vi "RXMux-Remote.vi"() -> ()   [LabVIEW 2009]
uses:
  <vilib>/NXT/Subs/LVHSConnector.ctl
  <vilib>/NXT/Block Support/NXT_InputPort.ctl
  <vilib>/NXT/Dual Mode Library/Display/drawNumber.vi
  <vilib>/NXT/Dual Mode Library/Display/drawText.vi
panel:
  in  "Channe to  Select":u8(ring) items=["Read Channel", "Select Ch1", "Select Ch2", "Select Ch3", "Select Ch4"]
  out "NXT dup":T1
  in  "Input Port":T2 items=["Port 1", "Port 2", "Port 3", "Port 4"]
  in  "stop":bool
  in  "NXT":T1
  # "mindsensors.com\nCopyright (c) 2009 by mindsensors.com\nEmail: info (<at>) mindsensors (<dot>) com\n\nThis program is free software. You can redistribute it and/or modify\nit under the terms of the GNU General Public License as published by\nthe Free Software Foundation; version 3 of the License.\nRead the license at: http://www.gnu.org/licenses/gpl.txt"
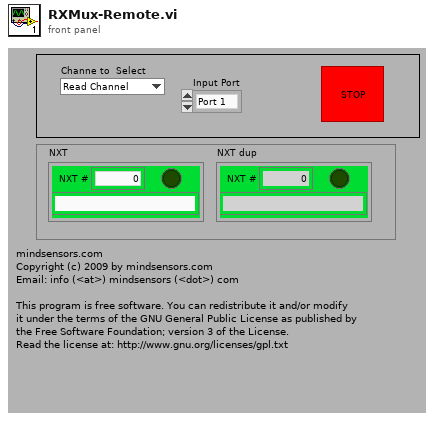
[diagram p1: front panel]
types:
  T1 = typedef "LVHSConnector.ctl" = cluster{"error":errorcluster, "address":string, "NXT #":i32, "Show Error":bool}
  T2 = typedef "NXT_InputPort.ctl" = u8
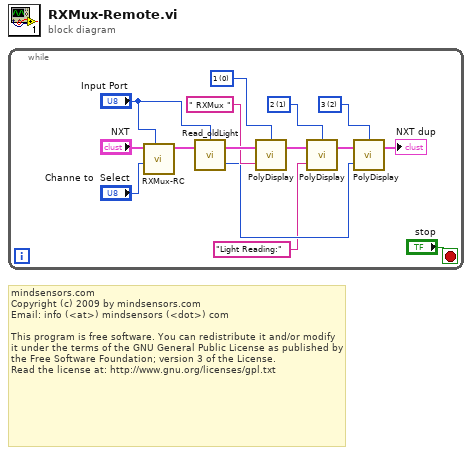
[diagram p0: block diagram]
diagram:
  # "mindsensors.com\nCopyright (c) 2009 by mindsensors.com\nEmail: info (<at>) mindsensors (<dot>) com\n\nThis program is free software. You can redistribute it and/or modify\nit under the terms of the GNU General Public License as published by\nthe Free Software Foundation; version 3 of the License.\nRead the license at: http://www.gnu.org/licenses/gpl.txt"
  n1 = while {
    stop <- "stop" stop-if-true
    w3 = i16 2 items=["1", "2", "3", "4", "5", "6", "7", "8"] ("Line")
    w8 = i16 1 items=["1", "2", "3", "4", "5", "6", "7", "8"] ("Line")
    w11 = i16 0 items=["1", "2", "3", "4", "5", "6", "7", "8"] ("Line")
    n2 = call "RXMux-RC.vi"("Input Port"="Input Port", "Channe to  Select"="Channe to  Select", "NXT"="NXT") -> ("NXT dup"=w14:T1)  [unwired: 7 in, 1 out]
    n3 = call <vilib>:"Read_oldLight.vi"("NXT"=w14, "Port (Port 3)"="Input Port") -> ("light"=w4:i16, "NXT"=w10:T1)  [unwired: 1 in]
    n4 = call-poly <vilib>:"PolyDisplay.vi"("Text"=" RXMux ", "NXT"=w10, "Line"=w11) -> ("NXT"=w7:T1)  [unwired: 1 in]
    n5 = call-poly <vilib>:"PolyDisplay.vi"("Text"="Light Reading:", "NXT"=w7, "Line"=w8) -> ("NXT"=w5:T1)  [unwired: 1 in]
    n6 = call-poly <vilib>:"PolyDisplay.vi"("number"=w4, "NXT"=w5, "Line"=w3) -> ("NXT"=→"NXT dup":T1)  [unwired: 1 in]
  }
